vi "Esophageal_VideoCaptureCard_Initialize.vi"(8 "error in (no error)":errorcluster) -> (0 "error out":errorcluster, 2 "Capture Card Image Out":T2, 3 "Capture Card Camera Out":T1 caption="FastHRME Camera Session Out")   [LabVIEW 2021]
uses:
  <vilib>/vision/Image Controls.llb/IMAQ Image.ctl
  <vilib>/userdefined/High Color/IMAQdx.ctl
  <vilib>/vision/driver/IMAQdx.llb/IMAQdx Acquisition Mode.ctl
  <vilib>/vision/driver/NI_Vision_Acquisition_Software.lvlib
panel:
  # "SubVI Inputs"
  # "SubVI Outputs"
  # "Mono"
  # "17301505"
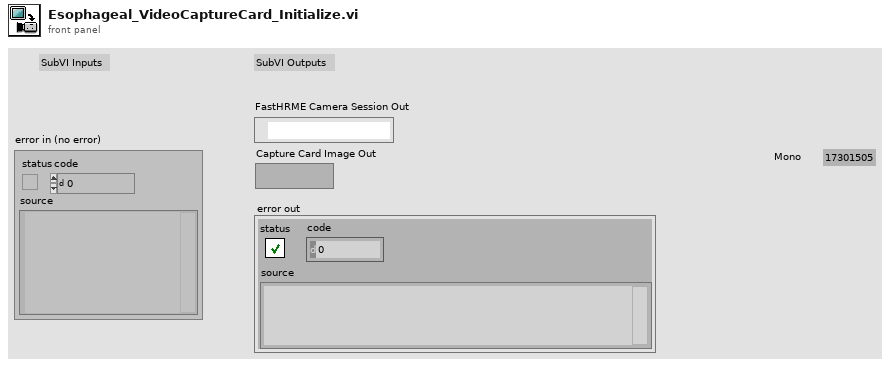
[diagram p1: front panel]
types:
  T1 = typedef "IMAQdx.ctl" = refnum<k21>
  T2 = typedef "IMAQ Image.ctl" = refnum<image>
  T3 = typedef "NI_Vision_Acquisition_Software.lvlib/IMAQdx Acquisition Mode.ctl" = enum32{"One Shot", "Continuous"}
  T4 = typedef "Image Type" = u32
  T5 = cluster{"Type":u32, "Version":u32, "Flags":u32, "SerialNumberHigh":u32, "SerialNumberLow":u32, "BusType":u32, "InterfaceName":string, "VendorName":string, "ModelName":string, "CameraFileName":string, "CameraAttributeURL":string}[]
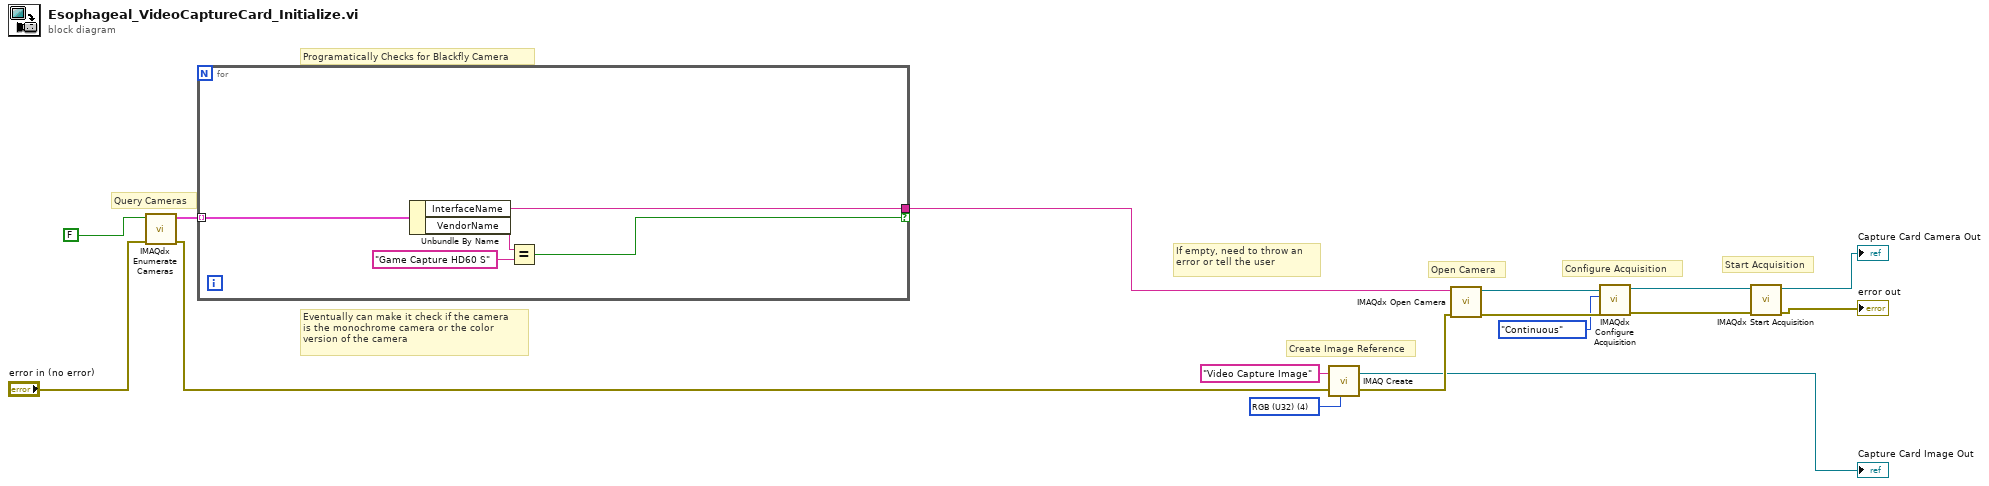
[diagram p0: block diagram]
diagram:
  w15 = T4 4 items=["Grayscale (U8)", "Grayscale (I16)", "Grayscale (SGL)", "Complex (CSG)", "RGB (U32)", "HSL (U32)", "RGB (U64)", "Grayscale (U16)"] ("Image Type")
  # "Eventually can make it check if the camera\nis the monochrome camera or the color\nversion of the camera"
  # "If empty, need to throw an error or tell the user"
  # "Query Cameras"
  # "Programatically Checks for Blackfly Camera"
  # "Start Acquisition"
  # "Configure Acquisition"
  # "Open Camera"
  # "Create Image Reference"
  n1 = call <vilib>:"IMAQdx Enumerate Cameras.vi"("error in"="error in (no error)", "Connected Only? (Yes)"=FALSE) -> ("error out"=w5:errorcluster, "Camera Information Array"=w7:T5)  [unwired: 8 in]
  n2 = for {
    tunnel: w7 -> [w21] mode=indexing
    tunnel: [w18] -> w2 if=w17
    n3 = Unbundle By Name(w21) -> ("InterfaceName"=w18:string, "VendorName"=w20:string)
    n4 = Equal?(x=w20, y="Game Capture HD60 S") -> (x = y?=w17:bool)
  }
  n5 = call "IMAQ Create"("Image Name"="Video Capture Image", "Image Type"=w15, "error in (no error)"=w5) -> ("New Image"=→"Capture Card Image Out":T2, "error out"=w9:errorcluster)  [unwired: 2 in]
  n6 = call <vilib>:"IMAQdx Open Camera.vi"("error in"=w9, "Session In"=w2) -> ("error out"=w13:errorcluster, "Session Out"=w14:T1)  [unwired: 8 in]
  n7 = call <vilib>:"IMAQdx Configure Acquisition.vi"("error in"=w13, "Continuous?"=IMAQdx_Acquisition_Mode."Continuous", "Session In"=w14) -> ("error out"=w10:errorcluster, "Session Out"=w11:T1)  [unwired: 7 in]
  n8 = call <vilib>:"IMAQdx Start Acquisition.vi"("error in"=w10, "Session In"=w11) -> ("error out"=→"error out":errorcluster, "Session Out"=→"Capture Card Camera Out":T1)  [unwired: 8 in]
